vi "Data Logging Save Config.vi"(8 "error in (no error)":errorcluster, 10 "Cluster":T1, 11 "Path":path) -> (0 "error out":errorcluster)   [LabVIEW 2014]
uses:
  TypeDef/Datalogger_State_SaveConfigFile.ctl
  <vilib>/Utility/config.llb/Write Key (String).vi
  <vilib>/Utility/config.llb/Write Key (U32).vi
  <vilib>/Utility/config.llb/Write Key (Path).vi
  <vilib>/Utility/config.llb/Write Key (Boolean).vi
  <vilib>/Utility/config.llb/NI_LVConfig.lvlib
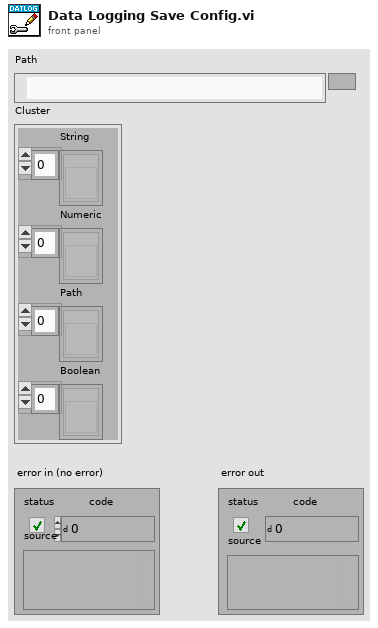
[diagram p1: front panel]
types:
  T1 = cluster{"String":refnum<vi>[], "Numeric":refnum<vi>[], "Path":refnum<vi>[], "Boolean":refnum<vi>[]}
  T2 = typedef "Datalogger_State_SaveConfigFile.ctl" = enum16{"Open File", "Item 1", "Item 2", "Item 3", "Item 4", "Close File"}
  T3 = typedef "NI_LVConfig.lvlib/Config Data RefNum.ctl" = refnum<k1>
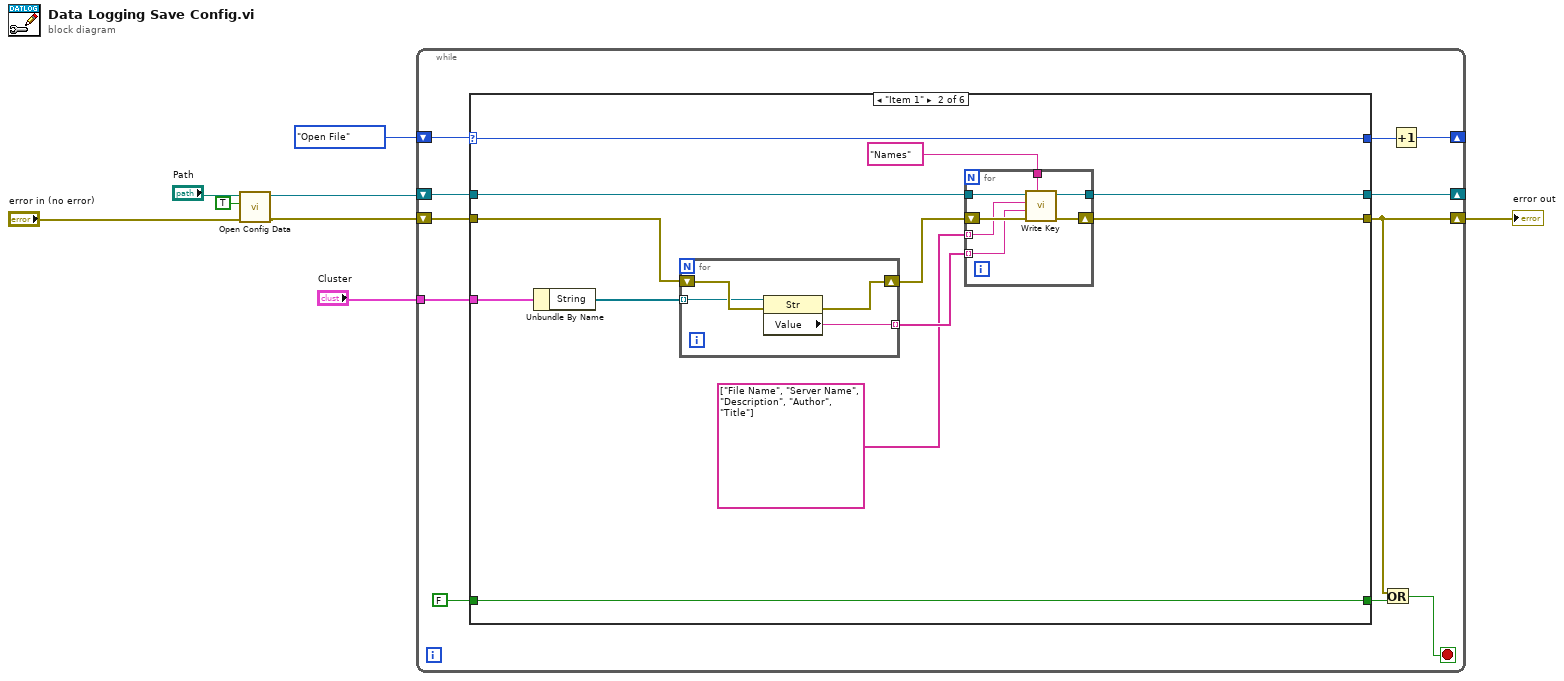
[diagram p0: block diagram]
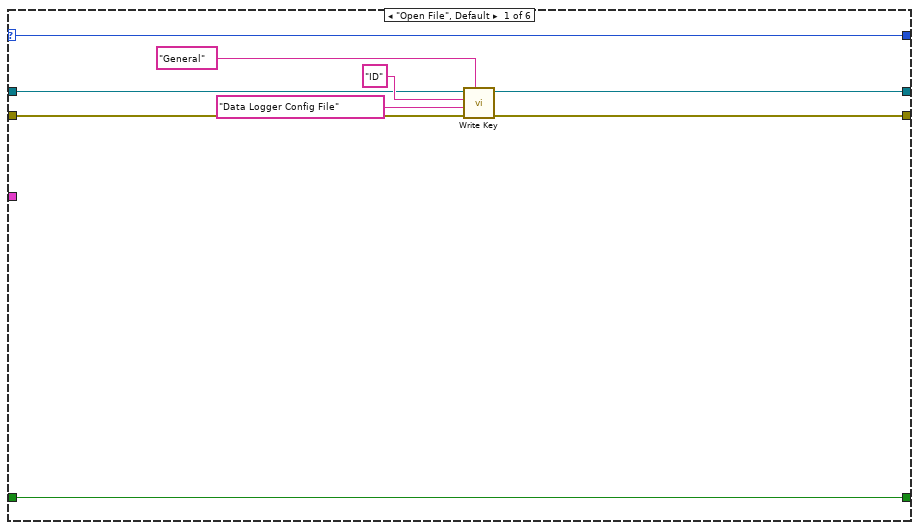
[diagram p2: hidden frame]
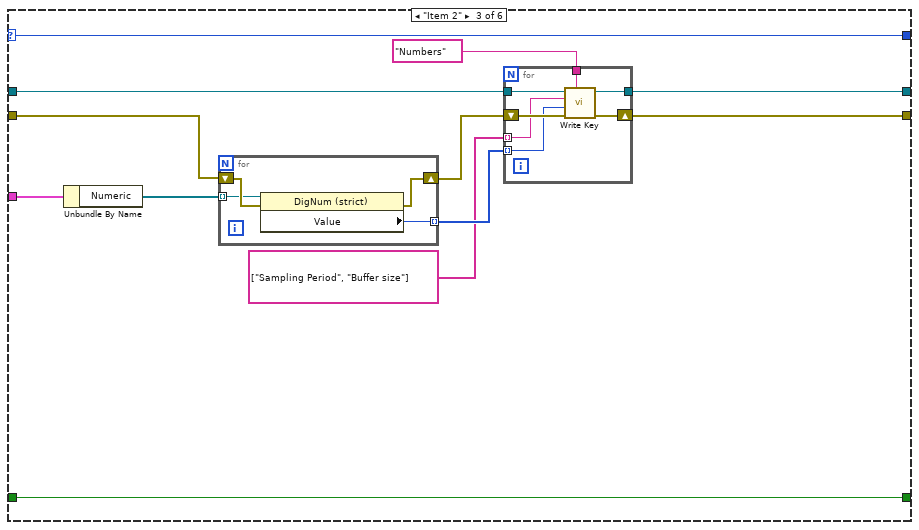
[diagram p3: hidden frame]
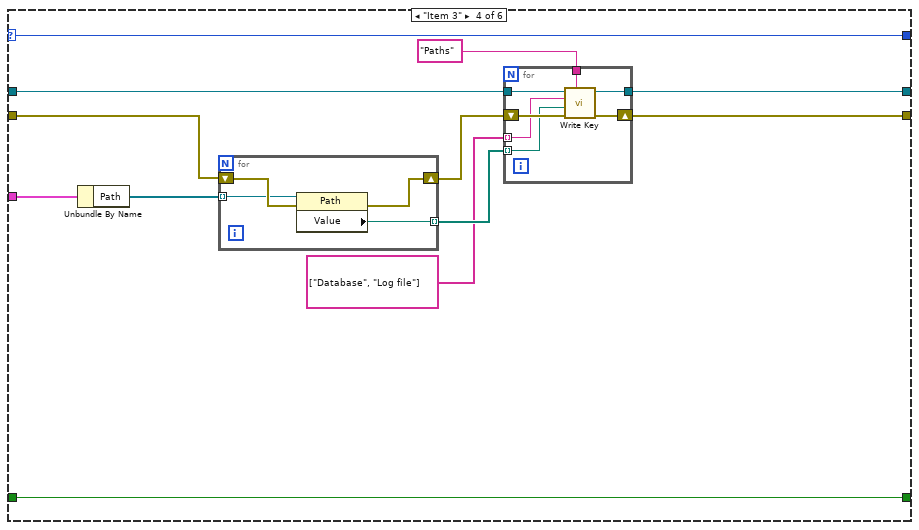
[diagram p4: hidden frame]
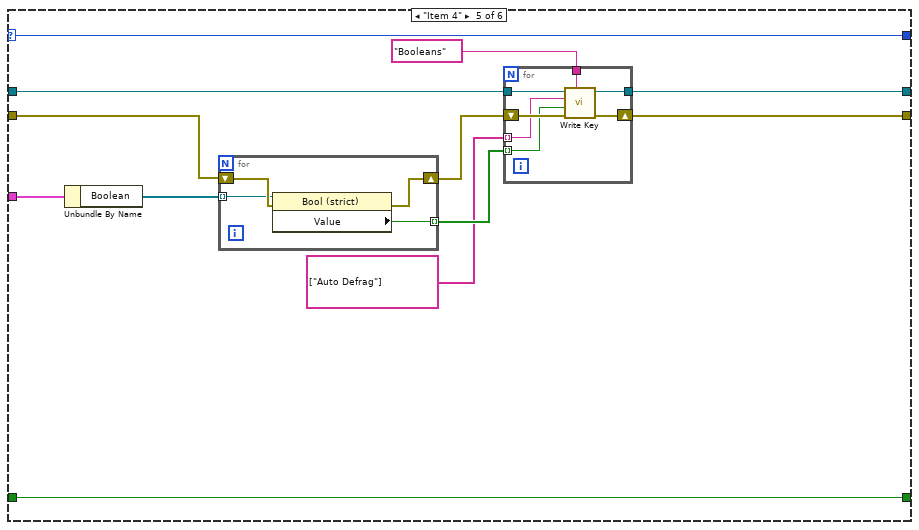
[diagram p5: hidden frame]
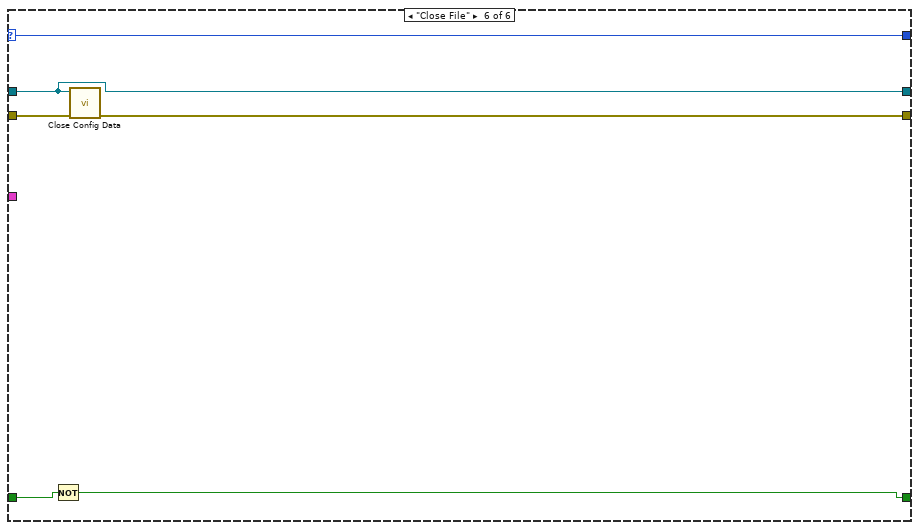
[diagram p6: hidden frame]
diagram:
  n1 = call <vilib>:"Open Config Data.vi"("error in (no error)"="error in (no error)", "create file if necessary (T)"=TRUE, "configuration file path"="Path") -> ("error out"=w4:errorcluster, "refnum"=w3:T3)  [unwired: 6 in, 1 out]
  n2 = while {
    shift-right: [w14] -> _
    shift-left: Datalogger_State_SaveConfigFile."Open File" -> [w19]
    tunnel: "Cluster" -> [w18]
    shift-right: [w9] -> w2
    shift-left: w4 -> [w17]
    shift-right: [w13] -> _
    shift-left: w3 -> [w16]
    stop <- w10 stop-if-true
    n3 = case shown="\"Item 1\"" w19 {
      selector: w19 -> [w24 w40 w63 w86 w109 w123]
      tunnel: w18 -> [_ w39 w62 w85 w108 _]
      tunnel: [w24 w40 w63 w86 w109 w123] -> w15
      tunnel: w17 -> [w22 w38 w61 w84 w107 w126]
      tunnel: [w21 w31 w54 w77 w100 w125] -> w9
      tunnel: [w20 w35 w58 w81 w104 w124] -> w13
      tunnel: w16 -> [w25 w36 w59 w82 w105 w124]
      tunnel: [w23 w30 w53 w76 w99 w121] -> w11
      tunnel: FALSE -> [w23 w30 w53 w76 w99 w122]
      frame "Open File", Default {
        n4 = call-poly <vilib>:"Write Key.vi"("section"="General", "error in (no error)"=w22, "value"="Data Logger Config File" ("section"), "key"="ID" ("section"), "refnum"=w25) -> ("error out"=w21:errorcluster, "refnum out"=w20:T3)  [unwired: 4 in, 1 out]
      }
      frame "Item 1" {
        n5 = Unbundle By Name(w39) -> ("String"=w37:refnum<vi>[])
        n6 = for {
          tunnel: [w51] -> w32 mode=indexing
          shift-right: [w49] -> w33
          shift-left: w38 -> [w50]
          tunnel: w37 -> [w48] mode=indexing
          n7 = property class="Str"(reference=w48, error in=w50) -> (error out=w49:errorcluster, "Value"=w51:string)  [unwired: 1 out]
        }
        n8 = for {
          tunnel: "Names" ("section") -> [w47]
          tunnel: w36 -> [w46]
          shift-right: [w44] -> w31
          shift-left: w33 -> [w45]
          tunnel: w32 -> [w43] mode=indexing
          tunnel: [w42] -> w35
          tunnel: string[] ["File Name", "Server Name", "Description", "Author", "Title"] -> [w41] mode=indexing
          n9 = call-poly <vilib>:"Write Key.vi"("section"=w47, "error in (no error)"=w45, "value"=w43, "key"=w41, "refnum"=w46) -> ("error out"=w44:errorcluster, "refnum out"=w42:T3)  [unwired: 4 in, 1 out]
        }
      }
      frame "Item 2" {
        n10 = Unbundle By Name(w62) -> ("Numeric"=w60:refnum<vi>[])
        n11 = for {
          tunnel: [w74] -> w55 mode=indexing
          shift-right: [w72] -> w56
          shift-left: w61 -> [w73]
          tunnel: w60 -> [w71] mode=indexing
          n12 = property class="DigNum (strict)"(reference=w71, error in=w73) -> (error out=w72:errorcluster, "Value"=w74:u32)  [unwired: 1 out]
        }
        n13 = for {
          tunnel: "Numbers" ("section") -> [w70]
          tunnel: w59 -> [w69]
          shift-right: [w67] -> w54
          shift-left: w56 -> [w68]
          tunnel: string[] ["Sampling Period", "Buffer size"] -> [w66] mode=indexing
          tunnel: w55 -> [w65] mode=indexing
          tunnel: [w64] -> w58
          n14 = call-poly <vilib>:"Write Key.vi"("section"=w70, "error in (no error)"=w68, "value"=w65, "key"=w66, "refnum"=w69) -> ("error out"=w67:errorcluster, "refnum out"=w64:T3)  [unwired: 4 in, 1 out]
        }
      }
      frame "Item 3" {
        n15 = Unbundle By Name(w85) -> ("Path"=w83:refnum<vi>[])
        n16 = for {
          tunnel: [w97] -> w78 mode=indexing
          shift-right: [w95] -> w79
          shift-left: w84 -> [w96]
          tunnel: w83 -> [w94] mode=indexing
          n17 = property class="Path"(reference=w94, error in=w96) -> (error out=w95:errorcluster, "Value"=w97:path)  [unwired: 1 out]
        }
        n18 = for {
          tunnel: "Paths" ("section") -> [w93]
          tunnel: w82 -> [w92]
          shift-right: [w90] -> w77
          shift-left: w79 -> [w91]
          tunnel: string[] ["Database", "Log file"] -> [w89] mode=indexing
          tunnel: w78 -> [w87] mode=indexing
          tunnel: [w88] -> w81
          n19 = call-poly <vilib>:"Write Key.vi"("section"=w93, "error in (no error)"=w91, "value"=w87, "key"=w89, "refnum"=w92) -> ("error out"=w90:errorcluster, "refnum out"=w88:T3)  [unwired: 4 in, 1 out]
        }
      }
      frame "Item 4" {
        n20 = Unbundle By Name(w108) -> ("Boolean"=w106:refnum<vi>[])
        n21 = for {
          tunnel: [w120] -> w101 mode=indexing
          shift-right: [w118] -> w102
          shift-left: w107 -> [w119]
          tunnel: w106 -> [w117] mode=indexing
          n22 = property class="Bool (strict)"(reference=w117, error in=w119) -> (error out=w118:errorcluster, "Value"=w120:bool)  [unwired: 1 out]
        }
        n23 = for {
          tunnel: "Booleans" ("section") -> [w116]
          tunnel: w105 -> [w115]
          shift-right: [w113] -> w100
          shift-left: w102 -> [w114]
          tunnel: string[] ["Auto Defrag"] -> [w112] mode=indexing
          tunnel: w101 -> [w110] mode=indexing
          tunnel: [w111] -> w104
          n24 = call-poly <vilib>:"Write Key.vi"("section"=w116, "error in (no error)"=w114, "value"=w110, "key"=w112, "refnum"=w115) -> ("error out"=w113:errorcluster, "refnum out"=w111:T3)  [unwired: 4 in, 1 out]
        }
      }
      frame "Close File" {
        n25 = Not(x=w122) -> (.not. x?=w121:bool)
        n26 = call <vilib>:"Close Config Data.vi"("error in (no error)"=w126, "refnum"=w124) -> ("error out"=w125:errorcluster)  [unwired: 8 in, 1 out]
      }
    }
    n27 = Or(x=w9, y=w11) -> (x .or. y?=w10:bool)
    n28 = Increment(x=w15) -> (x+1=w14:T2)
  }
  "error out" <- w2
